vi "DDS_Clock.vi"() -> ()   [LabVIEW 2016] (continued)
time[ms]"=7.7499999999999805, "f1 [Hz] CH0"=309000000.0}, {"total time[ms]"=7.79999999999998, "f1 [Hz] CH0"=308800000.0}, {"total time[ms]"=7.79999999999998, "f1 [Hz] CH0"=308800000.0}, {"total time[ms]"=7.84999999999998, "f1 [Hz] CH0"=308600000.0}, {"total time[ms]"=7.84999999999998, "f1 [Hz] CH0"=308600000.0}, {"total time[ms]"=7.89999999999998, "f1 [Hz] CH0"=308400000.0}, {"total time[ms]"=7.89999999999998, "f1 [Hz] CH0"=308400000.0}, {"total time[ms]"=7.94999999999998, "f1 [Hz] CH0"=308200000.0}, {"total time[ms]"=7.94999999999998, "f1 [Hz] CH0"=308200000.0}, {"total time[ms]"=7.99999999999998, "f1 [Hz] CH0"=308000000.0}, {"total time[ms]"=7.99999999999998, "f1 [Hz] CH0"=308000000.0}, {"total time[ms]"=8.04999999999998, "f1 [Hz] CH0"=307800000.0}, {"total time[ms]"=8.04999999999998, "f1 [Hz] CH0"=307800000.0}, {"total time[ms]"=8.09999999999998, "f1 [Hz] CH0"=307600000.0}, {"total time[ms]"=8.09999999999998, "f1 [Hz] CH0"=307600000.0}, {"total time[ms]"=8.14999999999998, "f1 [Hz] CH0"=307400000.0}, {"total time[ms]"=8.14999999999998, "f1 [Hz] CH0"=307400000.0}, {"total time[ms]"=8.199999999999982, "f1 [Hz] CH0"=307200000.0}, {"total time[ms]"=8.199999999999982, "f1 [Hz] CH0"=307200000.0}, {"total time[ms]"=8.249999999999982, "f1 [Hz] CH0"=307000000.0}, {"total time[ms]"=8.249999999999982, "f1 [Hz] CH0"=307000000.0}, {"total time[ms]"=8.299999999999983, "f1 [Hz] CH0"=306800000.0}, {"total time[ms]"=8.299999999999983, "f1 [Hz] CH0"=306800000.0}, {"total time[ms]"=8.349999999999984, "f1 [Hz] CH0"=306600000.0}, {"total time[ms]"=8.349999999999984, "f1 [Hz] CH0"=306600000.0}, {"total time[ms]"=8.399999999999984, "f1 [Hz] CH0"=306400000.0}, {"total time[ms]"=8.399999999999984, "f1 [Hz] CH0"=306400000.0}, {"total time[ms]"=8.449999999999985, "f1 [Hz] CH0"=306200000.0}, {"total time[ms]"=8.449999999999985, "f1 [Hz] CH0"=306200000.0}, {"total time[ms]"=8.499999999999986, "f1 [Hz] CH0"=306000000.0}, {"total time[ms]"=8.499999999999986, "f1 [Hz] CH0"=306000000.0}, {"total time[ms]"=8.549999999999986, "f1 [Hz] CH0"=305800000.0}, {"total time[ms]"=8.549999999999986, "f1 [Hz] CH0"=305800000.0}, {"total time[ms]"=8.599999999999987, "f1 [Hz] CH0"=305600000.0}, {"total time[ms]"=8.599999999999987, "f1 [Hz] CH0"=305600000.0}, {"total time[ms]"=8.649999999999988, "f1 [Hz] CH0"=305400000.0}, {"total time[ms]"=8.649999999999988, "f1 [Hz] CH0"=305400000.0}, {"total time[ms]"=8.699999999999989, "f1 [Hz] CH0"=305200000.0}, {"total time[ms]"=8.699999999999989, "f1 [Hz] CH0"=305200000.0}, {"total time[ms]"=8.74999999999999, "f1 [Hz] CH0"=305000000.0}, {"total time[ms]"=8.74999999999999, "f1 [Hz] CH0"=305000000.0}, {"total time[ms]"=8.79999999999999, "f1 [Hz] CH0"=304800000.0}, {"total time[ms]"=8.79999999999999, "f1 [Hz] CH0"=304800000.0}, {"total time[ms]"=8.84999999999999, "f1 [Hz] CH0"=304600000.0}, {"total time[ms]"=8.84999999999999, "f1 [Hz] CH0"=304600000.0}, {"total time[ms]"=8.899999999999991, "f1 [Hz] CH0"=304400000.0}, {"total time[ms]"=8.899999999999991, "f1 [Hz] CH0"=304400000.0}, {"total time[ms]"=8.949999999999992, "f1 [Hz] CH0"=304200000.0}, {"total time[ms]"=8.949999999999992, "f1 [Hz] CH0"=304200000.0}, {"total time[ms]"=8.999999999999993, "f1 [Hz] CH0"=304000000.0}, {"total time[ms]"=8.999999999999993, "f1 [Hz] CH0"=304000000.0}, {"total time[ms]"=9.049999999999994, "f1 [Hz] CH0"=303800000.0}, {"total time[ms]"=9.049999999999994, "f1 [Hz] CH0"=303800000.0}, {"total time[ms]"=9.099999999999994, "f1 [Hz] CH0"=303600000.0}, {"total time[ms]"=9.099999999999994, "f1 [Hz] CH0"=303600000.0}, {"total time[ms]"=9.149999999999995, "f1 [Hz] CH0"=303400000.0}, {"total time[ms]"=9.149999999999995, "f1 [Hz] CH0"=303400000.0}, {"total time[ms]"=9.199999999999996, "f1 [Hz] CH0"=303200000.0}, {"total time[ms]"=9.199999999999996, "f1 [Hz] CH0"=303200000.0}, {"total time[ms]"=9.249999999999996, "f1 [Hz] CH0"=303000000.0}, {"total time[ms]"=9.249999999999996, "f1 [Hz] CH0"=303000000.0}, {"total time[ms]"=9.299999999999997, "f1 [Hz] CH0"=302800000.0}, {"total time[ms]"=9.299999999999997, "f1 [Hz] CH0"=302800000.0}, {"total time[ms]"=9.349999999999998, "f1 [Hz] CH0"=302600000.0}, {"total time[ms]"=9.349999999999998, "f1 [Hz] CH0"=302600000.0}, {"total time[ms]"=9.399999999999999, "f1 [Hz] CH0"=302400000.0}, {"total time[ms]"=9.399999999999999, "f1 [Hz] CH0"=302400000.0}, {"total time[ms]"=9.45, "f1 [Hz] CH0"=302200000.0}, {"total time[ms]"=9.45, "f1 [Hz] CH0"=302200000.0}, {"total time[ms]"=9.5, "f1 [Hz] CH0"=302000000.0}, {"total time[ms]"=9.5, "f1 [Hz] CH0"=302000000.0}, {"total time[ms]"=9.55, "f1 [Hz] CH0"=301800000.0}, {"total time[ms]"=9.55, "f1 [Hz] CH0"=301800000.0}, {"total time[ms]"=9.600000000000001, "f1 [Hz] CH0"=301600000.0}, {"total time[ms]"=9.600000000000001, "f1 [Hz] CH0"=301600000.0}, {"total time[ms]"=9.650000000000002, "f1 [Hz] CH0"=301400000.0}, {"total time[ms]"=9.650000000000002, "f1 [Hz] CH0"=301400000.0}, {"total time[ms]"=9.700000000000003, "f1 [Hz] CH0"=301200000.0}, {"total time[ms]"=9.700000000000003, "f1 [Hz] CH0"=301200000.0}, {"total time[ms]"=9.750000000000004, "f1 [Hz] CH0"=301000000.0}, {"total time[ms]"=9.750000000000004, "f1 [Hz] CH0"=301000000.0}, {"total time[ms]"=9.800000000000004, "f1 [Hz] CH0"=300800000.0}, {"total time[ms]"=9.800000000000004, "f1 [Hz] CH0"=300800000.0}, {"total time[ms]"=9.850000000000005, "f1 [Hz] CH0"=300600000.0}, {"total time[ms]"=9.850000000000005, "f1 [Hz] CH0"=300600000.0}, {"total time[ms]"=9.900000000000006, "f1 [Hz] CH0"=300400000.0}, {"total time[ms]"=9.900000000000006, "f1 [Hz] CH0"=300400000.0}, {"total time[ms]"=9.950000000000006, "f1 [Hz] CH0"=300200000.0}, {"total time[ms]"=9.950000000000006, "f1 [Hz] CH0"=300200000.0}, {"total time[ms]"=10.000000000000007, "f1 [Hz] CH0"=300000000.0}, {"total time[ms]"=10.000000000000007, "f1 [Hz] CH0"=300000000.0}, {"total time[ms]"=10.050000000000008, "f1 [Hz] CH0"=300200000.0}, {"total time[ms]"=10.050000000000008, "f1 [Hz] CH0"=300200000.0}, {"total time[ms]"=10.100000000000009, "f1 [Hz] CH0"=300400000.0}, {"total time[ms]"=10.100000000000009, "f1 [Hz] CH0"=300400000.0}, {"total time[ms]"=10.15000000000001, "f1 [Hz] CH0"=300600000.0}, {"total time[ms]"=10.15000000000001, "f1 [Hz] CH0"=300600000.0}, {"total time[ms]"=10.20000000000001, "f1 [Hz] CH0"=300800000.0}, {"total time[ms]"=10.20000000000001, "f1 [Hz] CH0"=300800000.0}, {"total time[ms]"=10.25000000000001, "f1 [Hz] CH0"=301000000.0}, {"total time[ms]"=10.25000000000001, "f1 [Hz] CH0"=301000000.0}, {"total time[ms]"=10.300000000000011, "f1 [Hz] CH0"=301200000.0}, {"total time[ms]"=10.300000000000011, "f1 [Hz] CH0"=301200000.0}, {"total time[ms]"=10.350000000000012, "f1 [Hz] CH0"=301400000.0}, {"total time[ms]"=10.350000000000012, "f1 [Hz] CH0"=301400000.0}, {"total time[ms]"=10.400000000000013, "f1 [Hz] CH0"=301600000.0}, {"total time[ms]"=10.400000000000013, "f1 [Hz] CH0"=301600000.0}, {"total time[ms]"=10.450000000000014, "f1 [Hz] CH0"=301800000.0}, {"total time[ms]"=10.450000000000014, "f1 [Hz] CH0"=301800000.0}, {"total time[ms]"=10.500000000000014, "f1 [Hz] CH0"=302000000.0}, {"total time[ms]"=10.500000000000014, "f1 [Hz] CH0"=302000000.0}, {"total time[ms]"=10.550000000000015, "f1 [Hz] CH0"=302200000.0}, {"total time[ms]"=10.550000000000015, "f1 [Hz] CH0"=302200000.0}, {"total time[ms]"=10.600000000000016, "f1 [Hz] CH0"=302400000.0}, {"total time[ms]"=10.600000000000016, "f1 [Hz] CH0"=302400000.0}, {"total time[ms]"=10.650000000000016, "f1 [Hz] CH0"=302600000.0}, {"total time[ms]"=10.650000000000016, "f1 [Hz] CH0"=302600000.0}, {"total time[ms]"=10.700000000000017, "f1 [Hz] CH0"=302800000.0}, {"total time[ms]"=10.700000000000017, "f1 [Hz] CH0"=302800000.0}, {"total time[ms]"=10.750000000000018, "f1 [Hz] CH0"=303000000.0}, {"total time[ms]"=10.750000000000018, "f1 [Hz] CH0"=303000000.0}, {"total time[ms]"=10.800000000000018, "f1 [Hz] CH0"=303200000.0}, {"total time[ms]"=10.800000000000018, "f1 [Hz] CH0"=303200000.0}, {"total time[ms]"=10.85000000000002, "f1 [Hz] CH0"=303400000.0}, {"total time[ms]"=10.85000000000002, "f1 [Hz] CH0"=303400000.0}, {"total time[ms]"=10.90000000000002, "f1 [Hz] CH0"=303600000.0}, {"total time[ms]"=10.90000000000002, "f1 [Hz] CH0"=303600000.0}, {"total time[ms]"=10.95000000000002, "f1 [Hz] CH0"=303800000.0}, {"total time[ms]"=10.95000000000002, "f1 [Hz] CH0"=303800000.0}, {"total time[ms]"=11.000000000000021, "f1 [Hz] CH0"=304000000.0}, {"total time[ms]"=11.000000000000021, "f1 [Hz] CH0"=304000000.0}, {"total time[ms]"=11.050000000000022, "f1 [Hz] CH0"=304200000.0}, {"total time[ms]"=11.050000000000022, "f1 [Hz] CH0"=304200000.0}, {"total time[ms]"=11.100000000000023, "f1 [Hz] CH0"=304400000.0}, {"total time[ms]"=11.100000000000023, "f1 [Hz] CH0"=304400000.0}, {"total time[ms]"=11.150000000000023, "f1 [Hz] CH0"=304600000.0}, {"total time[ms]"=11.150000000000023, "f1 [Hz] CH0"=304600000.0}, {"total time[ms]"=11.200000000000024, "f1 [Hz] CH0"=304800000.0}, {"total time[ms]"=11.200000000000024, "f1 [Hz] CH0"=304800000.0}, {"total time[ms]"=11.250000000000025, "f1 [Hz] CH0"=305000000.0}, {"total time[ms]"=11.250000000000025, "f1 [Hz] CH0"=305000000.0}, {"total time[ms]"=11.300000000000026, "f1 [Hz] CH0"=305200000.0}, {"total time[ms]"=11.300000000000026, "f1 [Hz] CH0"=305200000.0}, {"total time[ms]"=11.350000000000026, "f1 [Hz] CH0"=305400000.0}, {"total time[ms]"=11.350000000000026, "f1 [Hz] CH0"=305400000.0}, {"total time[ms]"=11.400000000000027, "f1 [Hz] CH0"=305600000.0}, {"total time[ms]"=11.400000000000027, "f1 [Hz] CH0"=305600000.0}, {"total time[ms]"=11.450000000000028, "f1 [Hz] CH0"=305800000.0}, {"total time[ms]"=11.450000000000028, "f1 [Hz] CH0"=305800000.0}, {"total time[ms]"=11.500000000000028, "f1 [Hz] CH0"=306000000.0}, {"total time[ms]"=11.500000000000028, "f1 [Hz] CH0"=306000000.0}, {"total time[ms]"=11.55000000000003, "f1 [Hz] CH0"=306200000.0}, {"total time[ms]"=11.55000000000003, "f1 [Hz] CH0"=306200000.0}, {"total time[ms]"=11.60000000000003, "f1 [Hz] CH0"=306400000.0}, {"total time[ms]"=11.60000000000003, "f1 [Hz] CH0"=306400000.0}, {"total time[ms]"=11.65000000000003, "f1 [Hz] CH0"=306600000.0}, {"total time[ms]"=11.65000000000003, "f1 [Hz] CH0"=306600000.0}, {"total time[ms]"=11.700000000000031, "f1 [Hz] CH0"=306800000.0}, {"total time[ms]"=11.700000000000031, "f1 [Hz] CH0"=306800000.0}, {"total time[ms]"=11.750000000000032, "f1 [Hz] CH0"=307000000.0}, {"total time[ms]"=11.750000000000032, "f1 [Hz] CH0"=307000000.0}, {"total time[ms]"=11.800000000000033, "f1 [Hz] CH0"=307200000.0}, {"total time[ms]"=11.800000000000033, "f1 [Hz] CH0"=307200000.0}, {"total time[ms]"=11.850000000000033, "f1 [Hz] CH0"=307400000.0}, {"total time[ms]"=11.850000000000033, "f1 [Hz] CH0"=307400000.0}, {"total time[ms]"=11.900000000000034, "f1 [Hz] CH0"=307600000.0}, {"total time[ms]"=11.900000000000034, "f1 [Hz] CH0"=307600000.0}, {"total time[ms]"=11.950000000000035, "f1 [Hz] CH0"=307800000.0}, {"total time[ms]"=11.950000000000035, "f1 [Hz] CH0"=307800000.0}, {"total time[ms]"=12.000000000000036, "f1 [Hz] CH0"=308000000.0}, {"total time[ms]"=12.000000000000036, "f1 [Hz] CH0"=308000000.0}, {"total time[ms]"=12.050000000000036, "f1 [Hz] CH0"=308200000.0}, {"total time[ms]"=12.050000000000036, "f1 [Hz] CH0"=308200000.0}, {"total time[ms]"=12.100000000000037, "f1 [Hz] CH0"=308400000.0}, {"total time[ms]"=12.100000000000037, "f1 [Hz] CH0"=308400000.0}, {"total time[ms]"=12.150000000000038, "f1 [Hz] CH0"=308600000.0}, {"total time[ms]"=12.150000000000038, "f1 [Hz] CH0"=308600000.0}, {"total time[ms]"=12.200000000000038, "f1 [Hz] CH0"=308800000.0}, {"total time[ms]"=12.200000000000038, "f1 [Hz] CH0"=308800000.0}, {"total time[ms]"=12.250000000000039, "f1 [Hz] CH0"=309000000.0}, {"total time[ms]"=12.250000000000039, "f1 [Hz] CH0"=309000000.0}, {"total time[ms]"=12.30000000000004, "f1 [Hz] CH0"=309200000.0}, {"total time[ms]"=12.30000000000004, "f1 [Hz] CH0"=309200000.0}, {"total time[ms]"=12.35000000000004, "f1 [Hz] CH0"=309400000.0}, {"total time[ms]"=12.35000000000004, "f1 [Hz] CH0"=309400000.0}, {"total time[ms]"=12.400000000000041, "f1 [Hz] CH0"=309600000.0}, {"total time[ms]"=12.400000000000041, "f1 [Hz] CH0"=309600000.0}, {"total time[ms]"=12.450000000000042, "f1 [Hz] CH0"=309800000.0}, {"total time[ms]"=12.450000000000042, "f1 [Hz] CH0"=309800000.0}, {"total time[ms]"=12.500000000000043, "f1 [Hz] CH0"=310000000.0}, {"total time[ms]"=12.500000000000043, "f1 [Hz] CH0"=310000000.0}, {"total time[ms]"=12.550000000000043, "f1 [Hz] CH0"=310200000.0}, {"total time[ms]"=12.550000000000043, "f1 [Hz] CH0"=310200000.0}, {"total time[ms]"=12.600000000000044, "f1 [Hz] CH0"=310400000.0}, {"total time[ms]"=12.600000000000044, "f1 [Hz] CH0"=310400000.0}, {"total time[ms]"=12.650000000000045, "f1 [Hz] CH0"=310600000.0}, {"total time[ms]"=12.650000000000045, "f1 [Hz] CH0"=310600000.0}, {"total time[ms]"=12.700000000000045, "f1 [Hz] CH0"=310800000.0}, {"total time[ms]"=12.700000000000045, "f1 [Hz] CH0"=310800000.0}, {"total time[ms]"=12.750000000000046, "f1 [Hz] CH0"=311000000.0}, {"total time[ms]"=12.750000000000046, "f1 [Hz] CH0"=311000000.0}, {"total time[ms]"=12.800000000000047, "f1 [Hz] CH0"=311200000.0}, {"total time[ms]"=12.800000000000047, "f1 [Hz] CH0"=311200000.0}, {"total time[ms]"=12.850000000000048, "f1 [Hz] CH0"=311400000.0}, {"total time[ms]"=12.850000000000048, "f1 [Hz] CH0"=311400000.0}, {"total time[ms]"=12.900000000000048, "f1 [Hz] CH0"=311600000.0}, {"total time[ms]"=12.900000000000048, "f1 [Hz] CH0"=311600000.0}, {"total time[ms]"=12.950000000000049, "f1 [Hz] CH0"=311800000.0}, {"total time[ms]"=12.950000000000049, "f1 [Hz] CH0"=311800000.0}, {"total time[ms]"=13.00000000000005, "f1 [Hz] CH0"=312000000.0}, {"total time[ms]"=13.00000000000005, "f1 [Hz] CH0"=312000000.0}, {"total time[ms]"=13.05000000000005, "f1 [Hz] CH0"=312200000.0}, {"total time[ms]"=13.05000000000005, "f1 [Hz] CH0"=312200000.0}, {"total time[ms]"=13.100000000000051, "f1 [Hz] CH0"=312400000.0}, {"total time[ms]"=13.100000000000051, "f1 [Hz] CH0"=312400000.0}, {"total time[ms]"=13.150000000000052, "f1 [Hz] CH0"=312600000.0}, {"total time[ms]"=13.150000000000052, "f1 [Hz] CH0"=312600000.0}, {"total time[ms]"=13.200000000000053, "f1 [Hz] CH0"=312800000.0}, {"total time[ms]"=13.200000000000053, "f1 [Hz] CH0"=312800000.0}, {"total time[ms]"=13.250000000000053, "f1 [Hz] CH0"=313000000.0}, {"total time[ms]"=13.250000000000053, "f1 [Hz] CH0"=313000000.0}, {"total time[ms]"=13.300000000000054, "f1 [Hz] CH0"=313200000.0}, {"total time[ms]"=13.300000000000054, "f1 [Hz] CH0"=313200000.0}, {"total time[ms]"=13.350000000000055, "f1 [Hz] CH0"=313400000.0}, {"total time[ms]"=13.350000000000055, "f1 [Hz] CH0"=313400000.0}, {"total time[ms]"=13.400000000000055, "f1 [Hz] CH0"=313600000.0}, {"total time[ms]"=13.400000000000055, "f1 [Hz] CH0"=313600000.0}, {"total time[ms]"=13.450000000000056, "f1 [Hz] CH0"=313800000.0}, {"total time[ms]"=13.450000000000056, "f1 [Hz] CH0"=313800000.0}, {"total time[ms]"=13.500000000000057, "f1 [Hz] CH0"=314000000.0}, {"total time[ms]"=13.500000000000057, "f1 [Hz] CH0"=314000000.0}, {"total time[ms]"=13.550000000000058, "f1 [Hz] CH0"=314200000.0}, {"total time[ms]"=13.550000000000058, "f1 [Hz] CH0"=314200000.0}, {"total time[ms]"=13.600000000000058, "f1 [Hz] CH0"=314400000.0}, {"total time[ms]"=13.600000000000058, "f1 [Hz] CH0"=314400000.0}, {"total time[ms]"=13.650000000000059, "f1 [Hz] CH0"=314600000.0}, {"total time[ms]"=13.650000000000059, "f1 [Hz] CH0"=314600000.0}, {"total time[ms]"=13.70000000000006, "f1 [Hz] CH0"=314800000.0}, {"total time[ms]"=13.70000000000006, "f1 [Hz] CH0"=314800000.0}, {"total time[ms]"=13.75000000000006, "f1 [Hz] CH0"=315000000.0}, {"total time[ms]"=13.75000000000006, "f1 [Hz] CH0"=315000000.0}, {"total time[ms]"=13.800000000000061, "f1 [Hz] CH0"=315200000.0}, {"total time[ms]"=13.800000000000061, "f1 [Hz] CH0"=315200000.0}, {"total time[ms]"=13.850000000000062, "f1 [Hz] CH0"=315400000.0}, {"total time[ms]"=13.850000000000062, "f1 [Hz] CH0"=315400000.0}, {"total time[ms]"=13.900000000000063, "f1 [Hz] CH0"=315600000.0}, {"total time[ms]"=13.900000000000063, "f1 [Hz] CH0"=315600000.0}, {"total time[ms]"=13.950000000000063, "f1 [Hz] CH0"=315800000.0}, {"total time[ms]"=13.950000000000063, "f1 [Hz] CH0"=315800000.0}, {"total time[ms]"=14.000000000000064, "f1 [Hz] CH0"=316000000.0}, {"total time[ms]"=14.000000000000064, "f1 [Hz] CH0"=316000000.0}, {"total time[ms]"=14.050000000000065, "f1 [Hz] CH0"=316200000.0}, {"total time[ms]"=14.050000000000065, "f1 [Hz] CH0"=316200000.0}, {"total time[ms]"=14.100000000000065, "f1 [Hz] CH0"=316400000.0}, {"total time[ms]"=14.100000000000065, "f1 [Hz] CH0"=316400000.0}, {"total time[ms]"=14.150000000000066, "f1 [Hz] CH0"=316600000.0}, {"total time[ms]"=14.150000000000066, "f1 [Hz] CH0"=316600000.0}, {"total time[ms]"=14.200000000000067, "f1 [Hz] CH0"=316800000.0}, {"total time[ms]"=14.200000000000067, "f1 [Hz] CH0"=316800000.0}, {"total time[ms]"=14.250000000000068, "f1 [Hz] CH0"=317000000.0}, {"total time[ms]"=14.250000000000068, "f1 [Hz] CH0"=317000000.0}, {"total time[ms]"=14.300000000000068, "f1 [Hz] CH0"=317200000.0}, {"total time[ms]"=14.300000000000068, "f1 [Hz] CH0"=317200000.0}, {"total time[ms]"=14.350000000000069, "f1 [Hz] CH0"=317400000.0}, {"total time[ms]"=14.350000000000069, "f1 [Hz] CH0"=317400000.0}, {"total time[ms]"=14.40000000000007, "f1 [Hz] CH0"=317600000.0}, {"total time[ms]"=14.40000000000007, "f1 [Hz] CH0"=317600000.0}, {"total time[ms]"=14.45000000000007, "f1 [Hz] CH0"=317800000.0}, {"total time[ms]"=14.45000000000007, "f1 [Hz] CH0"=317800000.0}, {"total time[ms]"=14.500000000000071, "f1 [Hz] CH0"=318000000.0}, {"total time[ms]"=14.500000000000071, "f1 [Hz] CH0"=318000000.0}, {"total time[ms]"=14.550000000000072, "f1 [Hz] CH0"=318200000.0}, {"total time[ms]"=14.550000000000072, "f1 [Hz] CH0"=318200000.0}, {"total time[ms]"=14.600000000000072, "f1 [Hz] CH0"=318400000.0}, {"total time[ms]"=14.600000000000072, "f1 [Hz] CH0"=318400000.0}, {"total time[ms]"=14.650000000000073, "f1 [Hz] CH0"=318600000.0}, {"total time[ms]"=14.650000000000073, "f1 [Hz] CH0"=318600000.0}, {"total time[ms]"=14.700000000000074, "f1 [Hz] CH0"=318800000.0}, {"total time[ms]"=14.700000000000074, "f1 [Hz] CH0"=318800000.0}, {"total time[ms]"=14.750000000000075, "f1 [Hz] CH0"=319000000.0}, {"total time[ms]"=14.750000000000075, "f1 [Hz] CH0"=319000000.0}, {"total time[ms]"=14.800000000000075, "f1 [Hz] CH0"=319200000.0}, {"total time[ms]"=14.800000000000075, "f1 [Hz] CH0"=319200000.0}, {"total time[ms]"=14.850000000000076, "f1 [Hz] CH0"=319400000.0}, {"total time[ms]"=14.850000000000076, "f1 [Hz] CH0"=319400000.0}, {"total time[ms]"=14.900000000000077, "f1 [Hz] CH0"=319600000.0}, {"total time[ms]"=14.900000000000077, "f1 [Hz] CH0"=319600000.0}, {"total time[ms]"=14.950000000000077, "f1 [Hz] CH0"=319800000.0}, {"total time[ms]"=14.950000000000077, "f1 [Hz] CH0"=319800000.0}, {"total time[ms]"=15.000000000000078, "f1 [Hz] CH0"=320000000.0}, {"total time[ms]"=15.000000000000078, "f1 [Hz] CH0"=320000000.0}, {"total time[ms]"=15.050000000000079, "f1 [Hz] CH0"=319800000.0}, {"total time[ms]"=15.050000000000079, "f1 [Hz] CH0"=319800000.0}, {"total time[ms]"=15.10000000000008, "f1 [Hz] CH0"=319600000.0}, {"total time[ms]"=15.10000000000008, "f1 [Hz] CH0"=319600000.0}, {"total time[ms]"=15.15000000000008, "f1 [Hz] CH0"=319400000.0}, {"total time[ms]"=15.15000000000008, "f1 [Hz] CH0"=319400000.0}, {"total time[ms]"=15.200000000000081, "f1 [Hz] CH0"=319200000.0}, {"total time[ms]"=15.200000000000081, "f1 [Hz] CH0"=319200000.0}, {"total time[ms]"=15.250000000000082, "f1 [Hz] CH0"=319000000.0}, {"total time[ms]"=15.250000000000082, "f1 [Hz] CH0"=319000000.0}, {"total time[ms]"=15.300000000000082, "f1 [Hz] CH0"=318800000.0}, {"total time[ms]"=15.300000000000082, "f1 [Hz] CH0"=318800000.0}, {"total time[ms]"=15.350000000000083, "f1 [Hz] CH0"=318600000.0}, {"total time[ms]"=15.350000000000083, "f1 [Hz] CH0"=318600000.0}, {"total time[ms]"=15.400000000000084, "f1 [Hz] CH0"=318400000.0}, {"total time[ms]"=15.400000000000084, "f1 
